vi "Set scrollbar value.vi"(8 "error in (no error)":errorcluster, 10 "Scrollbar value":i32) -> (0 "error out":errorcluster)   [LabVIEW 2013]
uses:
  Globals/gl_Time series viewer globals.vi
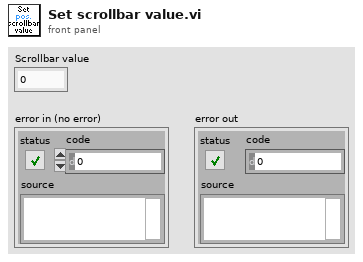
[diagram p1: front panel]
types:
  T1 = typedef "Timelapse viewer refs.ctl" = cluster{"This VI":refnum<vi>, "AVI Mode ind":refnum<vi>, "Play":refnum<vi>, "Stop":refnum<vi>, "Back":refnum<vi>, "Scrollbar":refnum<vi>, "Video length info":refnum<vi>, "Expected speed values":refnum<vi>, "Intensity":refnum<vi>, "Path":refnum<vi>, "Selection sliders":refnum<vi>, "Speed Graph ref":refnum<vi>, "Frame rate set (fps)":refnum<vi>}
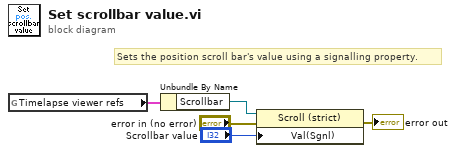
[diagram p0: block diagram]
diagram:
  # "Sets the position scroll bar's value using a signalling property."
  n1 = global read "gl_Time series viewer globals.vi" "Timelapse viewer refs"() -> (w4:T1)
  n2 = Unbundle By Name(w4) -> ("Scrollbar"=w3:refnum<vi>)
  n3 = property class="Scroll (strict)"(reference=w3, error in="error in (no error)", "Val(Sgnl)"="Scrollbar value") -> (error out=→"error out":errorcluster)  [unwired: 1 out]
